vi "标尺标定.vi"() -> ()   [LabVIEW 2018]
doc: "This example illustrates the use of the horizontal clamp tool. You can draw a region of inspection that contains at least two edges in the image. The VI measures the distance between the first and last edges."
uses:
  2658f9af-f960-436f-abe9-75b9ff3a2793.vi
  <vilib>/vision/NI_Vision_Development_Module.lvlib
panel:
  out "添加的数组":dbl[](array[numeric])
  in  "记录数据":bool
  in  "单次执行":bool
  in  "标尺方向选择":u16(ring) items=["横向放置", "竖向放置"]
  in  "标的值保存":bool
  in  "标尺间距单位":u16(ring)=3 items=["Undefined", "Angstr", "Micrometer", "Millimeter", "Centimeter", "Meter", "Kilometer", "Microinch", "Inch", "Feet", "Nautical miles", "Standardmiles", "Steps"]
  in  "标尺间距":dbl
  out "像素当量":sgl
  out "像素距离(pixels)":sgl
  out "图像显示":T1(plugin-control)
  in  "Stop":bool
  # "标尺标定"
  # "像素距离：两红线间距离，单位为像素\n像素当量：标尺间距/像素距离"
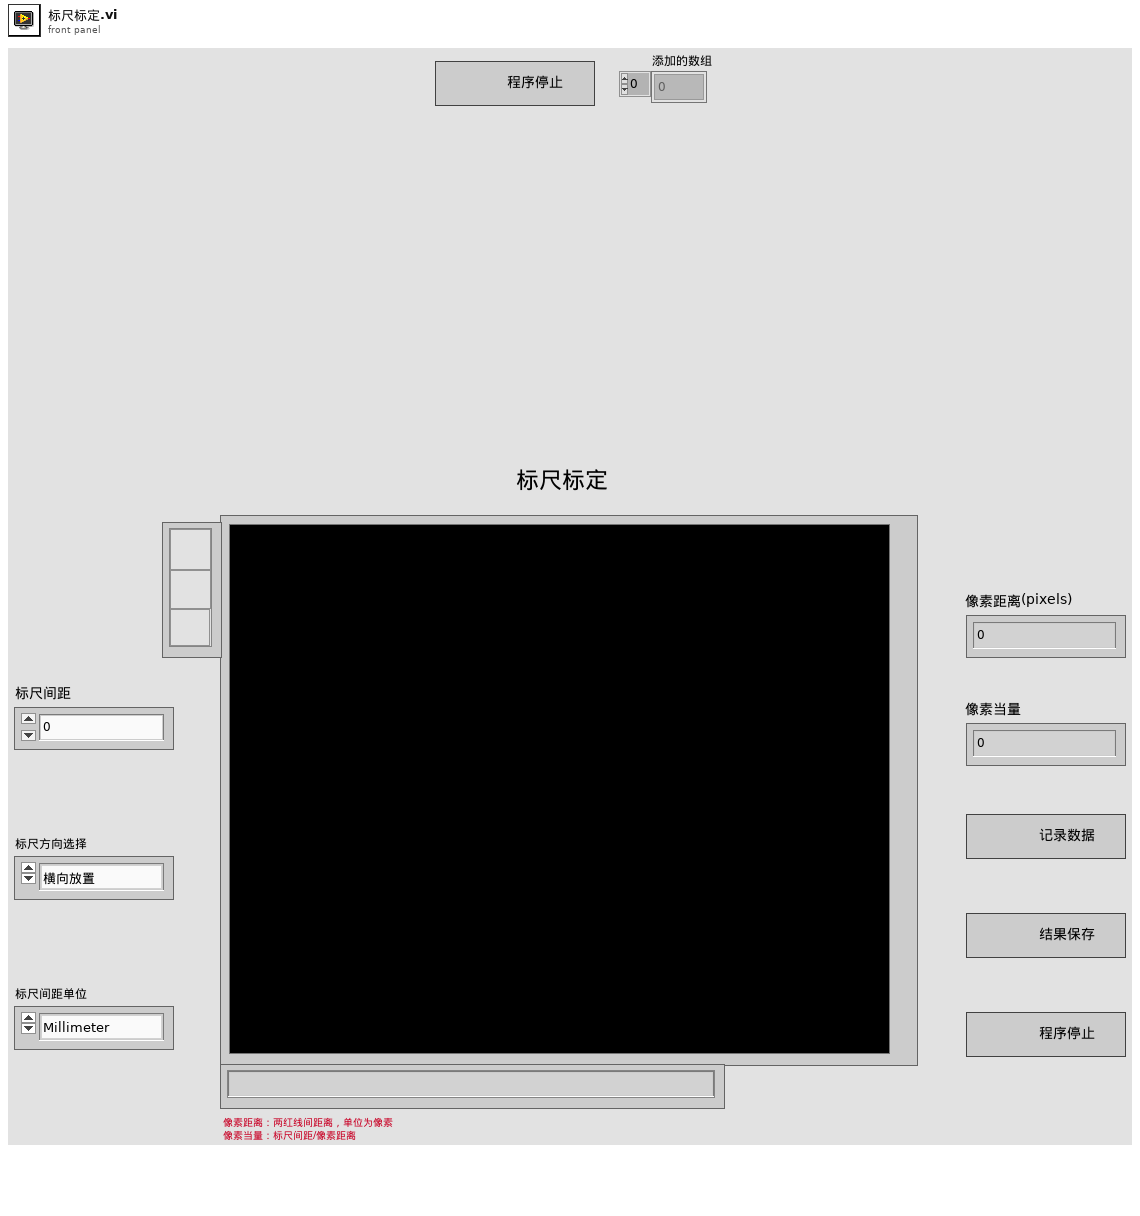
[diagram p1: front panel]
types:
  T1 = typedef "IMAQ Image.ctl" = refnum<image>
  T2 = enum8{"Enabled", "Disabled", "Disabled and Grayed Out"}
  T3 = enum32{"Invalid", "Standard", "Closed", "Hidden", "Minimized", "Maximized"}
  T4 = typedef "Image Type" = u32
  T5 = cluster{"Contrast":i32, "Filter width":i32, "Steepness":i32, "Subsampling Ratio":u32, "Show Search Area":bool, "Show Search Lines":bool, "Show Edges Found":bool, "Show Result":bool}
  T6 = cluster{"Global Rectangle":i32[], "Contours":cluster{"Contour Type":u32, "ROI Type":u32, "Points":i32[]}[]}
  T7 = typedef "IMAQ Rectangle" = cluster{"Left":i32, "Top":i32, "Right":i32, "Bottom":i32, "Rotation":dbl}
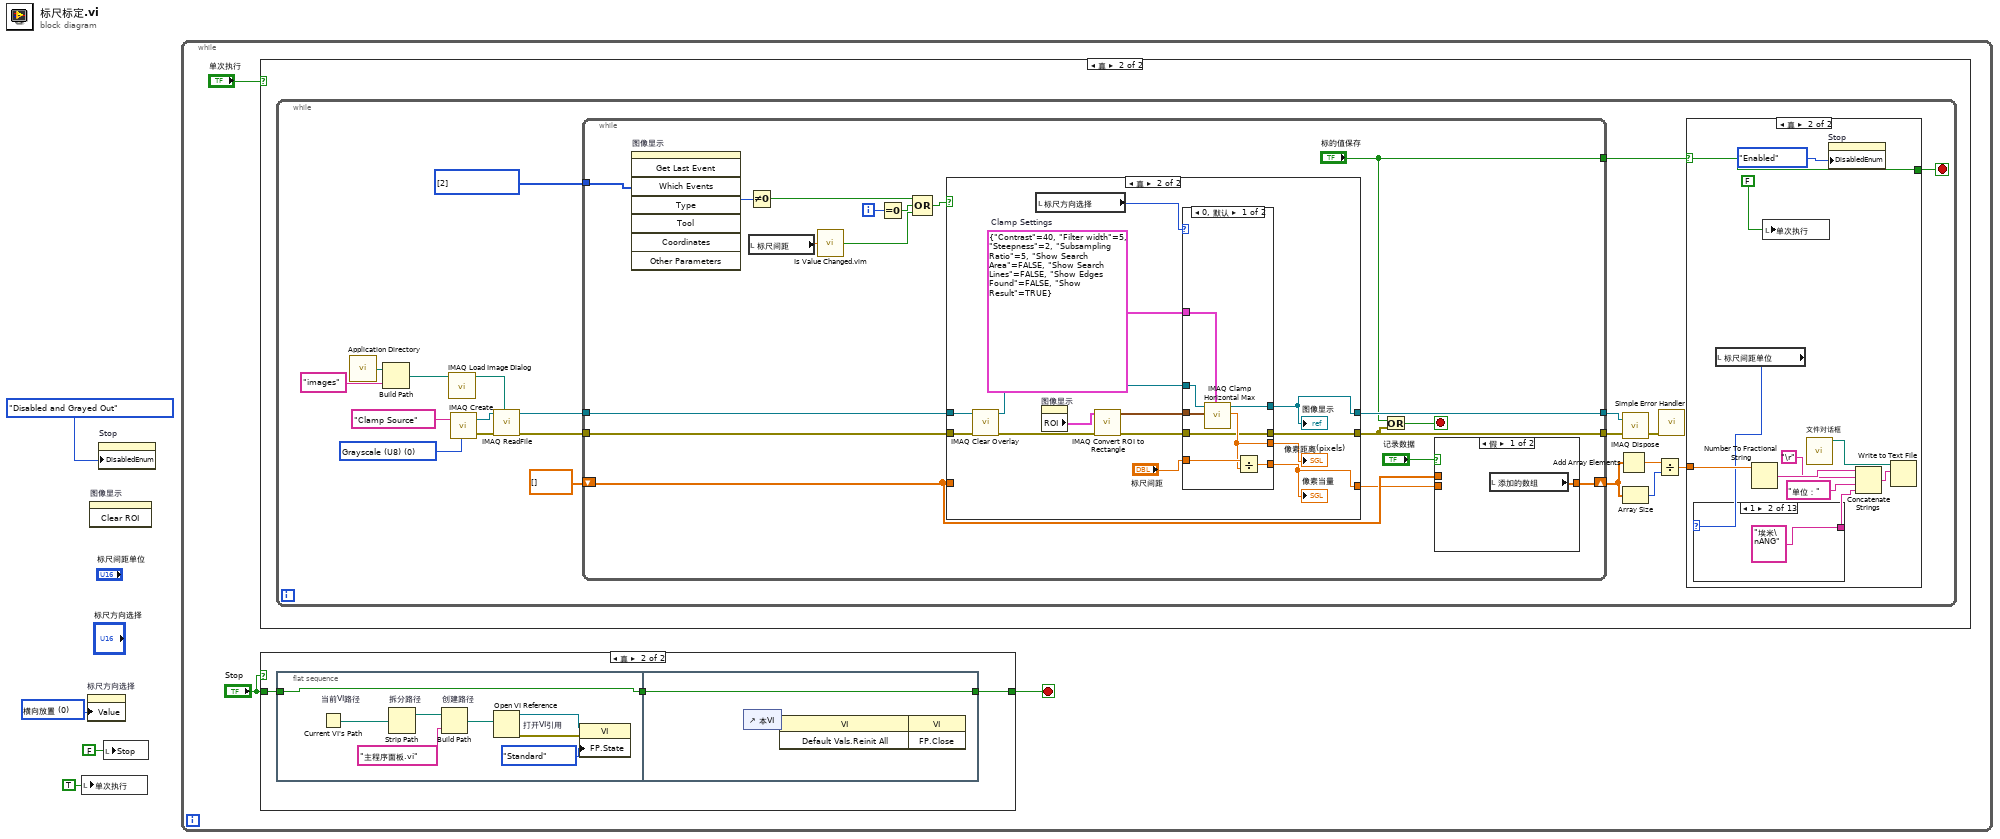
[diagram p0: block diagram]
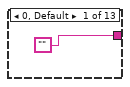
[diagram p4: hidden frame]
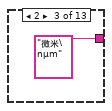
[diagram p5: hidden frame]
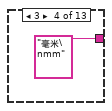
[diagram p6: hidden frame]
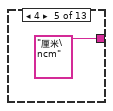
[diagram p7: hidden frame]
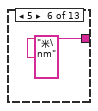
[diagram p8: hidden frame]
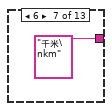
[diagram p9: hidden frame]
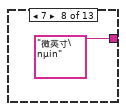
[diagram p10: hidden frame]
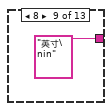
[diagram p11: hidden frame]
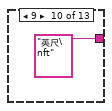
[diagram p12: hidden frame]
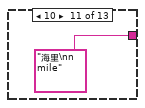
[diagram p13: hidden frame]
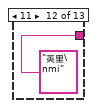
[diagram p14: hidden frame]
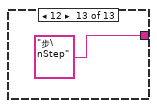
[diagram p15: hidden frame]
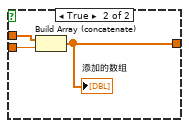
[diagram p16: hidden frame]
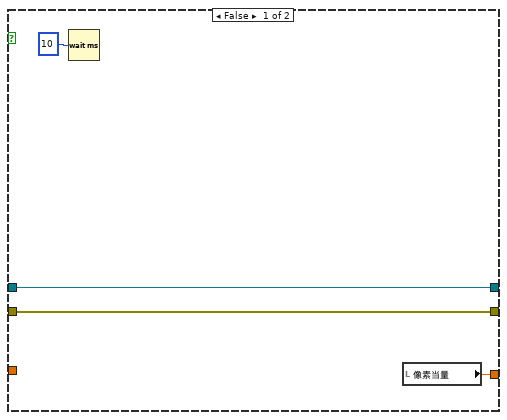
[diagram p17: hidden frame]
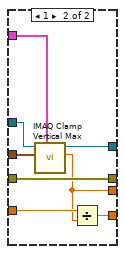
[diagram p18: hidden frame]
diagram:
  w3 = u16 0 items=["横向放置", "竖向放置"] ("标尺方向选择")
  n1 = local write "单次执行"(TRUE ("单次执行")) -> ()
  n2 = property on="标尺方向选择" class="Ring (严格)"("Value"=w3) -> ()  [unwired: 2 in, 2 out]
  n3 = invoke on="图像显示" class="ImageControl" method="Clear ROI"() -> ()  [unwired: 3 in, 3 out]
  n4 = property on="Stop" class="Bool (严格)"("DisabledEnum"=T2."Disabled and Grayed Out" ("禁用")) -> ()  [unwired: 2 in, 2 out]
  n5 = local write "Stop"(FALSE ("Stop")) -> ()
  n6 = while {
    stop <- w6 stop-if-true
    n7 = case shown="真" "单次执行" {
      frame False {
      }
      frame True {
        n8 = while {
          stop <- w8 stop-if-true
          w11 = i32[] [2] items=["No  event", "Click event", "Draw event", "Move event", "Size event", "Scroll event", "Activate event", "Close event", "Double click event"] ("Events list (all)")
          w15 = T4 0 items=["Grayscale (U8)", "Grayscale (I16)", "Grayscale (SGL)", "Complex (CSG)", "RGB (U32)", "HSL (U32)", "RGB (U64)", "Grayscale (U16)"] ("Image Type")
          n9 = call <vilib>:"Application Directory.vi"() -> ("Application Directory"=w20:path)
          n10 = Build Path(base path=w20, name or relative path="images") -> (appended path=w21:path)
          n11 = call "IMAQ Load Image Dialog"("Start Path"=w21) -> ("Path"=w19:path)  [unwired: 8 in, 2 out]
          n12 = call "IMAQ Create"("Image Name"="Clamp Source", "Image Type"=w15) -> ("New Image"=w17:T1, "error out"=w18:errorcluster)  [unwired: 3 in]
          n13 = call "IMAQ ReadFile"("File Path"=w19, "error in (no error)"=w18, "Image"=w17) -> ("error out"=w13:errorcluster, "Image Out"=w12:T1)  [unwired: 4 in, 3 out]
          n14 = while {
            tunnel: w12 -> [w70]
            tunnel: [w61] -> w27
            tunnel: [w68] -> w26
            tunnel: w13 -> [w67]
            tunnel: w11 -> [w66]
            tunnel: ["标的值保存"] -> w25
            shift-right: [w55] -> w10
            shift-left: dbl[] [] -> [w58]
            i -> [w65]
            stop <- w60 stop-if-true
            n15 = invoke on="图像显示" class="ImageControl" method="Get Last Event"("Which Events"=w66) -> ("Type"=w69:i32)  [unwired: 7 in, 7 out]
            n16 = Not Equal To 0?(x=w69) -> (x != 0?=w63:bool)
            n17 = local read "标尺间距"() -> (w54:dbl)
            n18 = call "Is Value Changed.vim"("value"=w54) -> ("changed or first call?"=w53:bool)
            n19 = Equal To 0?(x=w65) -> (x = 0?=w64:bool)
            n20 = Compound Arithmetic op=OR ("复合运算")(w63, w64, w53) -> (w62:bool)
            n21 = case shown="真" w62 {
              tunnel: w70 -> [w76 w89]
              tunnel: [w77 w92] -> w61
              tunnel: [w76 w91] -> w68
              tunnel: w67 -> [w77 w90]
              tunnel: w58 -> [_ _]
              tunnel: [w75 w79] -> w57
              frame False {
                n22 = Wait (ms)(milliseconds to wait=u32 10) -> ()  [unwired: 1 out]
                n23 = local read "像素当量"() -> (w75:sgl)
              }
              frame True {
                w83 = T5 {"Contrast"=40, "Filter width"=5, "Steepness"=2, "Subsampling Ratio"=5, "Show Search Area"=FALSE, "Show Search Lines"=FALSE, "Show Edges Found"=FALSE, "Show Result"=TRUE}  # Clamp Settings
                n24 = call "IMAQ Clear Overlay"("error in (no error)"=w90, "Image"=w89) -> ("error out"=w88:errorcluster, "Image Out"=w85:T1)  [unwired: 8 in]
                n25 = local read "标尺方向选择"() -> (w81:u16)
                n26 = property on="图像显示" class="ImageControl"() -> ("ROI"=w86:T6)  [unwired: 2 in, 2 out]
                n27 = call "IMAQ Convert ROI to Rectangle"("error in (no error)"=w88, "ROI Descriptor"=w86) -> ("error out"=w87:errorcluster, "Rectangle"=w84:T7)  [unwired: 7 in]
                n28 = case shown="0, 默认" w81 {
                  tunnel: [w93 w102] -> w92
                  tunnel: [w94 w104] -> w91
                  tunnel: w87 -> [w93 w102]
                  tunnel: w85 -> [w100 w103]
                  tunnel: w84 -> [w99 w108]
                  tunnel: w83 -> [w98 w107]
                  tunnel: "标尺间距" -> [w97 w106]
                  tunnel: [w95 w105] -> w79
                  tunnel: [w96 w101] -> w80
                  frame 0, Default {
                    n29 = call "IMAQ Clamp Horizontal Max"("Settings"=w98, "Rectangle"=w99, "Image"=w100) -> ("Distance"=w96:sgl, "Image Out"=w94:T1)  [unwired: 4 in, 3 out]
                    n30 = Divide(x=w97, y=w96) -> (x/y=w95:dbl)
                  }
                  frame 1 {
                    n31 = call "IMAQ Clamp Vertical Max"("Settings"=w107, "Rectangle"=w108, "Image"=w103) -> ("Distance"=w101:sgl, "Image Out"=w104:T1)  [unwired: 4 in, 3 out]
                    n32 = Divide(x=w106, y=w101) -> (x/y=w105:dbl)
                  }
                }
                "图像显示" <- w91
                "像素距离(pixels)" <- w80
                "像素当量" <- w79
              }
            }
            n33 = Or(x="标的值保存", y=w61) -> (x .or. y?=w60:bool)
            n34 = case shown="假" "记录数据" {
              tunnel: w58 -> [_ w74]
              tunnel: [w71 w73] -> w55
              tunnel: w57 -> [_ w72]
              frame False {
                n35 = local read "添加的数组"() -> (w71:dbl[])
              }
              frame True {
                n36 = Build Array (concatenate)(w74, w72) -> (w73:dbl[])
                "添加的数组" <- w73
              }
            }
          }
          n37 = Add Array Elements(numeric array=w10) -> (sum=w24:dbl)
          n38 = call "IMAQ Dispose"("Image"=w26, "error in (no error)"=w27) -> ("error out"=w28:errorcluster)  [unwired: 4 in]
          n39 = Array Size(array=w10) -> (size(s)=w23:i32)
          n40 = Divide(x=w24, y=w23) -> (x/y=w22:dbl)
          n41 = call <vilib>:"Simple Error Handler.vi"("error in (no error)"=w28) -> ()  [unwired: 4 in, 5 out]
          n42 = case shown="真" w25 {
            selector: w25 -> [_ w37]
            tunnel: w22 -> [_ w38]
            tunnel: [_ w37] -> w8
            frame False {
            }
            frame True {
              n43 = local read "标尺间距单位"() -> (w32:u16)
              n44 = case shown="1" w32 {
                tunnel: ["" "埃米\nANG" ("字符串") "微米\nμm" ("字符串") "毫米\nmm" ("字符串") "厘米\ncm" ("字符串") "米\nm" ("字符串") "千米\nkm" ("字符串") "微英寸\nμin" ("字符串") "英寸\nin" ("字符串") "英尺\nft" ("字符串") "海里\nn mile" ("字符串") "英里\nmi" ("字符串") "步\nStep" ("字符串")] -> w30
                frame 0, Default {
                }
                frame 1 {
                }
                frame 2 {
                }
                frame 3 {
                }
                frame 4 {
                }
                frame 5 {
                }
                frame 6 {
                }
                frame 7 {
                }
                frame 8 {
                }
                frame 9 {
                }
                frame 10 {
                }
                frame 11 {
                }
                frame 12 {
                }
              }
              n45 = Number To Fractional String(number=w38) -> (F-format string=w34:string)  [unwired: 3 in]
              n46 = local write "单次执行"(FALSE ("单次执行")) -> ()
              n47 = call "文件对话框"() -> ("selected path"=w39:path)  [unwired: 12 in, 3 out]
              n48 = property on="Stop" class="Bool (严格)"("DisabledEnum"=T2."Enabled" ("禁用")) -> ()  [unwired: 2 in, 2 out]
              n49 = Concatenate Strings(w34, "\r", "单位：" ("字符串"), w30) -> (w33:string)
              n50 = Write to Text File(file (use dialog)=w39, text=w33) -> ()  [unwired: 2 in, 3 out]
            }
          }
        }
      }
    }
    n51 = case shown="真" "Stop" {
      tunnel: "Stop" -> [w109 w111]
      tunnel: [w109 w110] -> w6
      frame False {
      }
      frame True {
        n52 = flat-sequence {
          tunnel: w111 -> [w113]
          tunnel: [w113] -> w112
          tunnel: [w121] -> w110
          tunnel: w112 -> [w121]
          frame #0 {
            n53 = Current VI's Path "当前VI路径"() -> (path=w118:path)
            n54 = Strip Path "拆分路径"(path=w118) -> (stripped path=w120:path)  [unwired: 1 out]
            n55 = Build Path "创建路径"(base path=w120, name or relative path="主程序面板.vi" ("名称或相对路径")) -> (appended path=w119:path)
            n56 = Open VI Reference "打开VI引用"(vi path=w119) -> (vi reference=w117:refnum<vi>, error out=w116:errorcluster)  [unwired: 5 in]
            n57 = property class="VI"(reference=w117, error in=w116, "FP.State"=T3."Standard" ("前面板窗口:状态")) -> ()  [unwired: 2 out]
          }
          frame #1 {
            n58 = control-ref of="本VI"() -> (w122:refnum<vi>)
            n59 = invoke class="VI" method="Default Vals.Reinit All"(reference=w122) -> (reference out=w123:refnum<vi>, error out=w124:errorcluster)  [unwired: 2 in, 1 out]
            n60 = invoke class="VI" method="FP.Close"(reference=w123, error in=w124) -> ()  [unwired: 1 in, 3 out]
          }
        }
      }
    }
  }
